vi "Unserialize.vi"(6 "All Build Configs":string[](array[string]), 8 "error in (no error)":errorcluster, 9 "Serialization Version":string, 10 "XML Node":refnum<class "XML Node.lvclass">, 11 "ZIP Item in":refnum<class "ZIP Item.lvclass">) -> (0 "error out":errorcluster, 2 "Invalid Version?":bool, 3 "ZIP Item out":refnum<class "ZIP Item.lvclass">)   [LabVIEW 2019, in "ZIP.lvlib" / "ZIP Item.lvclass"]
uses:
  ZIP Item.lvclass
  libs/Solution.lvlibp/Solution/XML Reader/XML Node.lvclass
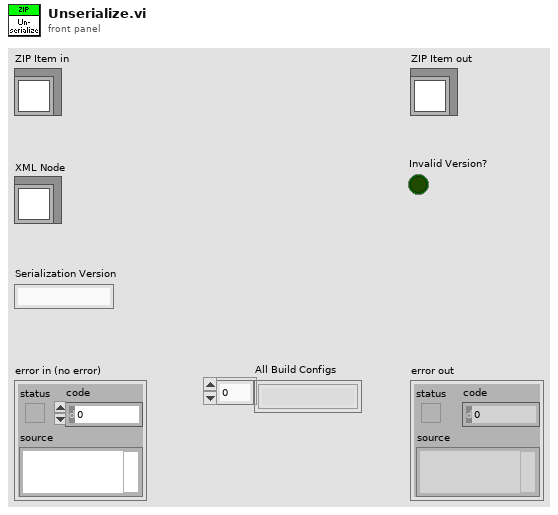
[diagram p1: front panel]
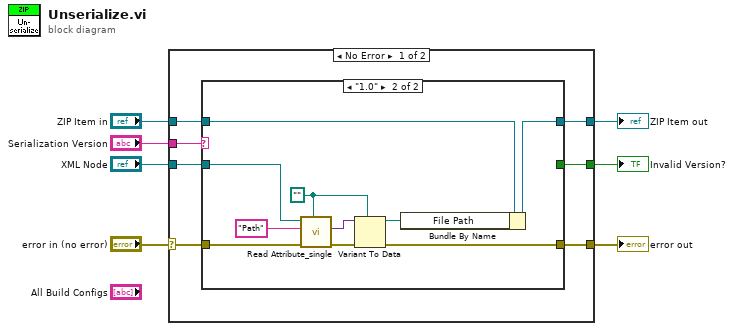
[diagram p0: block diagram]
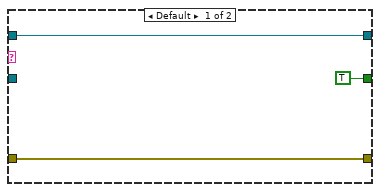
[diagram p2: hidden frame]
diagram:
  n1 = case shown="No Error" "error in (no error)" {
    selector: "error in (no error)" -> [w14 w28]
    tunnel: "XML Node" -> [w13 _]
    tunnel: [w12 w28] -> w5
    tunnel: "ZIP Item in" -> [w11 w29]
    tunnel: [w10 w29] -> w3
    tunnel: "Serialization Version" -> [w9 _]
    tunnel: [w8 _] -> w1
    frame No Error {
      n2 = case shown="\"1.0\"" w9 {
        tunnel: w14 -> [w15 w27]
        tunnel: w13 -> [_ w25]
        tunnel: [w15 w23] -> w12
        tunnel: w11 -> [w17 w20]
        tunnel: [w17 w19] -> w10
        tunnel: [TRUE _] -> w8
        frame Default {
        }
        frame "1.0" {
          w21 = path ""
          n3 = call "Read Attribute_single.vi"("Type"=w21, "error in (no error)"=w27, "Name"="Path", "XML Reader in"=w25) -> ("error out"=w26:errorcluster, "Value"=w22:variant)  [unwired: 6 in]
          n4 = Variant To Data(error in=w26, type=w21, Variant=w22) -> (data=w18:path, error out=w23:errorcluster)
          n5 = Bundle By Name(cluster=w20, "File Path"=w18) -> (w19:refnum<class "ZIP Item.lvclass">)
        }
      }
    }
    frame Error {
    }
  }
  "error out" <- w5
  "Invalid Version?" <- w1
  "ZIP Item out" <- w3
